vi "Load Teams.vi"() -> (2 "Names":string[](array[string]), 3 "Available Teams":refnum<class "Team.lvclass">[](array[class]))   [LabVIEW 2020, in "SB App.lvlib" / "SB App.lvclass"]
uses:
  SB App.lvclass
  SquareBattle/Team/Team.lvclass
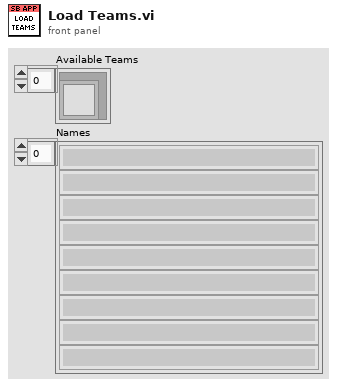
[diagram p1: front panel]
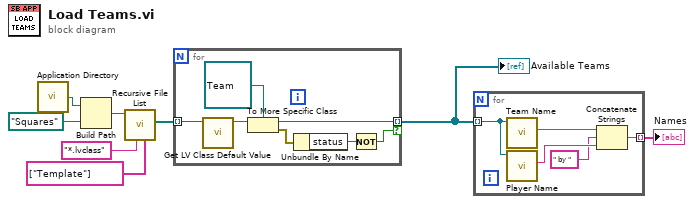
[diagram p0: block diagram]
diagram:
  n1 = call <vilib>:"Application Directory.vi"() -> ("Application Directory"=w8:path)
  n2 = Build Path(base path=w8, name or relative path=path "Squares") -> (appended path=w6:path)
  n3 = call <vilib>:"Recursive File List.vi"("Folders to Exclude"=string[] ["Template"], "pattern"="*.lvclass", "Folder Path"=w6) -> ("All Files in Dir"=w3:path[])  [unwired: 4 in, 4 out]
  n4 = for {
    tunnel: w3 -> [w15] mode=indexing
    tunnel: [w12] -> w2 mode=indexing if=w9
    n5 = call <vilib>:"Get LV Class Default Value.vi"("class path"=w15) -> ("object"=w14:refnum<class>)  [unwired: 9 in, 1 out]
    n6 = To More Specific Class(target class=refnum<class "Team.lvclass"> refnum ("SquareBattle:Team"), reference=w14) -> (specific class reference=w12:refnum<class "Team.lvclass">, error out=w11:errorcluster)  [unwired: 1 in]
    n7 = Unbundle By Name(w11) -> ("status"=w10:bool)
    n8 = Not(x=w10) -> (.not. x?=w9:bool)
  }
  "Available Teams" <- w2
  n9 = for {
    tunnel: w2 -> [w20] mode=indexing
    tunnel: [w16] -> w1 mode=indexing
    n10 = call-dynamic "Team Name.vi"("Team in"=w20) -> ("Team Name"=w19:string)  [unwired: 10 in]
    n11 = call-dynamic "Player Name.vi"("Team"=w20) -> ("Player Name"=w18:string)  [unwired: 10 in]
    n12 = Concatenate Strings(w19, " by " ("string"), w18) -> (w16:string)
  }
  "Names" <- w1
